vi "FTW-Connector-Ping.vi"(0 "FTW Actor Connector Type":refnum<class "FTW-Actor-Connector.lvclass">, 5 "Timeout":i32=100 format="%dmsec", 11 "error in":errorcluster) -> (4 "FTW Actor Connector":refnum<class "FTW-Actor-Connector.lvclass">, 6 "Timed out?":bool, 8 "Roundtrip Time":dbl format="%.6fsec", 15 "error out":errorcluster)   [LabVIEW 2013, in "FTW-Actor-Connector.lvclass"]
doc: "Performs a \"cold call\" to connect to a running Actor Instance at the given Instance Inbox Address. Normally, this method is wrapped by a \"Construct\" method in each specific Actor Connector subclass."
uses:
  FTW-Actor-Connector.lvclass
  FTW-Actor-Connector.lvclass/FTW-Actor-Connector.ctl
  socket/FTW-Socket.lvclass
panel:
  # "Inputs"
  # "Outputs"
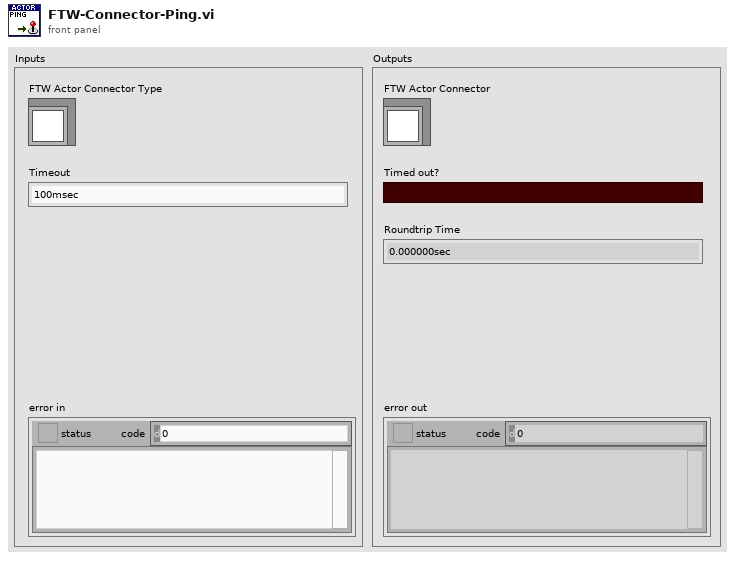
[diagram p1: front panel]
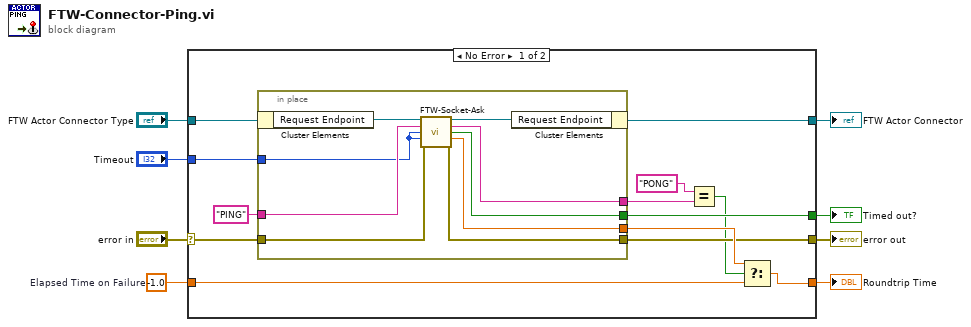
[diagram p0: block diagram]
diagram:
  w2 = -1.0  # Elapsed Time on Failure
  n1 = case shown="No Error" "error in" {
    selector: "error in" -> [w16 w32]
    tunnel: [w20 w33] -> w8
    tunnel: "FTW Actor Connector Type" -> [w21 w33]
    tunnel: [w11 w32] -> w5
    tunnel: "Timeout" -> [w19 _]
    tunnel: [w12 w31] -> w3
    tunnel: w2 -> [w9 w31]
    tunnel: [w17 _] -> w1
    frame No Error {
      n2 = in-place {
        in-place-border: w16 -> [w26]
        in-place-border: [w30] -> w11
        in-place-border: "PING" ("Request") -> [w25]
        in-place-border: w19 -> [w24]
        in-place-border: [w27] -> w15
        in-place-border: [w23] -> w17
        in-place-border: [w22] -> w13
        n3 = in-place-cluster #1(w21) -> ("Request Endpoint"=w29:refnum<class "FTW-Socket.lvclass">)
        n4 = call "FTW-Socket-Ask.vi"("FTW Socket"=w29, "Request"=w25, "Receive Timeout"=w24, "Send Timeout"=w24, "error in"=w26) -> ("FTW Socket out"=w28:refnum<class "FTW-Socket.lvclass">, "Response"=w27:string, "Timed out?"=w23:bool, "Roundtrip Time"=w22:dbl, "error out"=w30:errorcluster)  [unwired: 6 in]
        n5 = in-place-cluster #1("Request Endpoint"=w28) -> (w20:refnum<class "FTW-Actor-Connector.lvclass">)
      }
      n6 = Equal?(x="PONG", y=w15) -> (x = y?=w10:bool)
      n7 = Select(t=w13, s=w10, f=w9) -> (s? t:f=w12:dbl)
    }
    frame Error {
    }
  }
  "error out" <- w5
  "FTW Actor Connector" <- w8
  "Roundtrip Time" <- w3
  "Timed out?" <- w1
